vi "FPGA_I2C_Start.vi"(10 "Wait Time":u32, 11 "IO Cluster":T1) -> (2 "Done?":bool)   [LabVIEW 2020]
doc: "Sends the start bit on the data line to alert all slaves of upcoming transmission."
uses:
  Controls/FPGA_I2C IO Cluster.ctl
  Controls/FPGA I2C_Start State.ctl
  <vilib>/rvi/eio/common/nirviEmuTemplateMethod_errors.vi
  <vilib>/eio/EIOMethodNode/EIOMethodNode.xnode
  <vilib>/eio/EIONode/EIONode.xnode
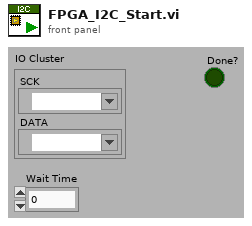
[diagram p1: front panel]
types:
  T1 = typedef "FPGA_I2C IO Cluster.ctl" = cluster{"SCK":refnum<k21>, "DATA":refnum<k21>}
  T2 = typedef "FPGA I2C_Start State.ctl" = enum16{"Set SCK High 1", "Wait 1", "Set DATA Low 1", "Wait 2", "Set SCK Low 1", "Wait 3", "Stop"}
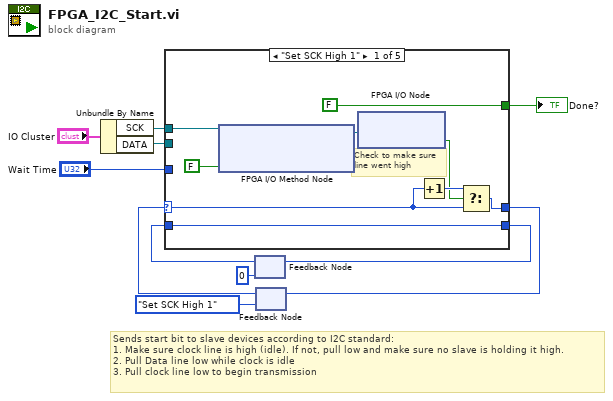
[diagram p0: block diagram]
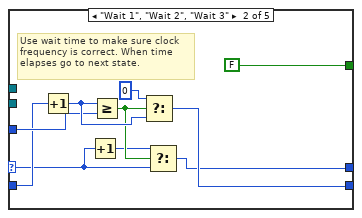
[diagram p2: hidden frame]
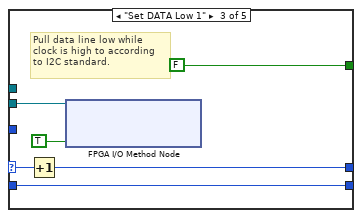
[diagram p3: hidden frame]
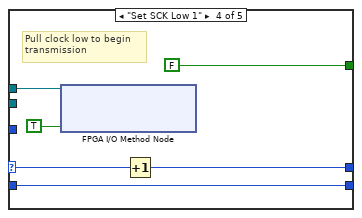
[diagram p4: hidden frame]
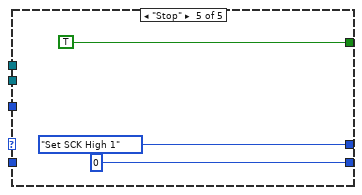
[diagram p5: hidden frame]
diagram:
  # "Sends start bit to slave devices according to I2C standard:\n1. Make sure clock line is high (idle). If not, pull low and make sure no slave is holding it high.\n2. Pull Data line low while clock is idle\n3. Pull clock line low to begin transmission"
  n1 = Unbundle By Name("IO Cluster") -> ("SCK"=w10:refnum<k21>, "DATA"=w11:refnum<k21>)
  n2 = feedback #1(u32 0 ("t")) -> (w6:u32)
  n3 = feedback #2(FPGA_I2C_Start_State."Set SCK High 1" ("Enum")) -> (w2:T2)
  n4 = case shown="\"Set SCK High 1\"" w2 {
    selector: w2 -> [w12 w22 w35 w41 _]
    tunnel: [FALSE FALSE FALSE FALSE TRUE] -> w4
    tunnel: "Wait Time" -> [_ w28 _ _ _]
    tunnel: [w19 w27 w33 w39 u32 0 ("t")] -> w5
    tunnel: w6 -> [w19 w26 w33 w39 _]
    tunnel: [w13 w23 w34 w40 FPGA_I2C_Start_State."Set SCK High 1" ("Enum")] -> w1
    tunnel: w10 -> [w18 _ _ w38 _]
    tunnel: w11 -> [_ _ w32 _ _]
    frame "Set SCK High 1" {
      # "Check to make sure line went high"
      n5 = xnode "FPGA I/O Method Node"("FPGA I/O In"=w18, "Enable"=FALSE) -> ("FPGA I/O Out"=w14:refnum<k21>)
      n6 = xnode "FPGA I/O Node"("FPGA I/O In"=w14) -> ("I/O Item"=w15:bool)  [unwired: 1 out]
      n7 = Increment(x=w12) -> (x+1=w16:T2)
      n8 = Select(t=w16, s=w15, f=w12) -> (s? t:f=w13:T2)
    }
    frame "Wait 1", "Wait 2", "Wait 3" {
      # "Use wait time to make sure clock\nfrequency is correct. When time\nelapses go to next state."
      n9 = Increment(x=w26) -> (x+1=w29:u32)
      n10 = Increment(x=w22) -> (x+1=w24:T2)
      n11 = Greater Or Equal?(x=w29, y=w28) -> (x >= y?=w25:bool)
      n12 = Select(t=u32 0, s=w25, f=w29) -> (s? t:f=w27:u32)
      n13 = Select(t=w24, s=w25, f=w22) -> (s? t:f=w23:T2)
    }
    frame "Set DATA Low 1" {
      # "Pull data line low while\nclock is high to according\nto I2C standard."
      n14 = Increment(x=w35) -> (x+1=w34:T2)
      n15 = xnode "FPGA I/O Method Node"("FPGA I/O In"=w32, "Enable"=TRUE) -> ()  [unwired: 1 out]
    }
    frame "Set SCK Low 1" {
      # "Pull clock low to begin\ntransmission"
      n16 = xnode "FPGA I/O Method Node"("FPGA I/O In"=w38, "Enable"=TRUE) -> ()  [unwired: 1 out]
      n17 = Increment(x=w41) -> (x+1=w40:T2)
    }
    frame "Stop" {
    }
  }
  "Done?" <- w4
  n18 = feedback-in #1(w5) -> ()
  n19 = feedback-in #2(w1) -> ()
